vi "Servo.vi"() -> ()   [LabVIEW 2020]
uses:
  <vilib>/MakerHub/LINX/Public/Utilities/Open Serial.vi
  <vilib>/MakerHub/LINX/Public/Sensors/Motion/Servo/Servo Open One Channel.vi
  <vilib>/MakerHub/LINX/Public/Sensors/Motion/Servo/Servo Close One Channel.vi
  <vilib>/MakerHub/LINX/LMH-LINX.lvlib
  <vilib>/MakerHub/LINX/Public/Sensors/Motion/Servo/Servo.lvlib
panel:
  out "Position":dbl
  in  "stop":bool
  in  "Turns":bool
  in  "Servo Channel":u8
  in  "Serial Port":refnum<visa-resource-name>="N/A"
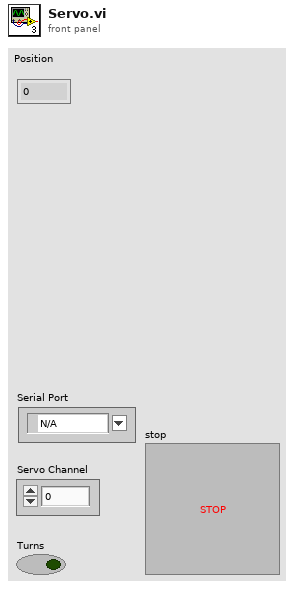
[diagram p1: front panel]
types:
  T1 = typedef "LMH-LINX.lvlib/LINX Ref.ctl" = cluster{"IO":T2, "Interface":T3, "LINX Device Config":T4}
  T2 = typedef "LMH-LINX.lvlib/Platform.ctl" = enum16{"Remote", "Local"}
  T3 = typedef "LMH-LINX.lvlib/Interface.ctl" = enum16{"Serial", "TCP"}
  T4 = typedef "LMH-LINX.lvlib/Device.lvlib/LINX Device Config.ctl" = cluster{"Interface":T3, "COM Port":refnum<visa-resource-name>, "TCP Configuration":T5, "Device Family":u8, "Device ID":u8, "Device Name":string, "TCP Ref":refnum<k5>, "Channels":T6}
  T5 = typedef "LMH-LINX.lvlib/Device.lvlib/TCP Config.ctl" = cluster{"IP Address":string, "Port":u16}
  T6 = typedef "LMH-LINX.lvlib/Channels.ctl" = cluster{"DI":u8[], "DO":u8[], "AI":u8[], "AO":u8[], "PWM":u8[], "QE":u8[], "UART":u8[], "I2C 2":u8[], "SPI":u8[], "CAN":u8[], "Servo":u8[], "AI Ref (V)":dbl, "AI Resolution (Bits)":u8, "AO Ref (V)":dbl, "AO Resolution (Bits)":u8}
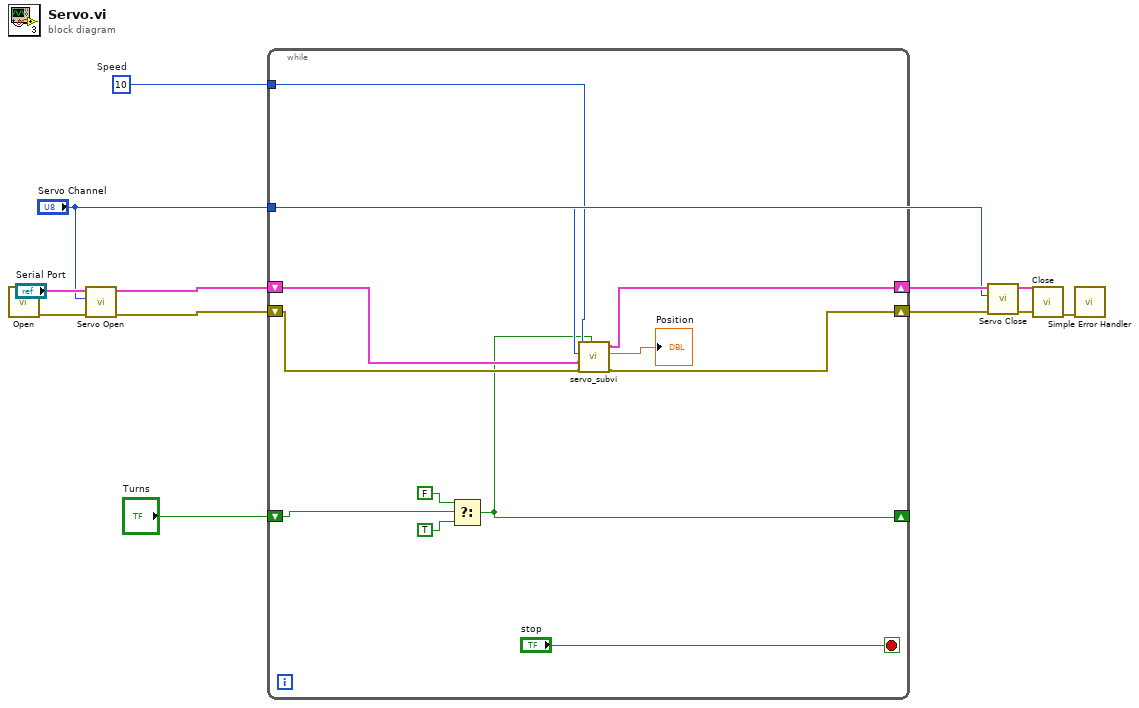
[diagram p0: block diagram]
diagram:
  w1 = u32 10  # Speed
  n1 = call-poly <vilib>:"Open.vi"("Serial Port"="Serial Port") -> ("Error Out"=w11:errorcluster, "LINX Resource"=w12:T1)  [unwired: 8 in, 1 out]
  n2 = call-poly <vilib>:"Servo Open.vi"("Error In"=w11, "Servo Channel"="Servo Channel", "LINX Resource"=w12) -> ("Error Out"=w6:errorcluster, "LINX Resource"=w7:T1)  [unwired: 7 in]
  n3 = while {
    tunnel: "Servo Channel" -> [w21]
    tunnel: w1 -> [w18]
    shift-right: [w22] -> w4
    shift-left: w7 -> [w25]
    shift-right: [w23] -> w5
    shift-left: w6 -> [w24]
    shift-right: [w16] -> _
    shift-left: "Turns" -> [w17]
    stop <- "stop" stop-if-true
    n4 = Select(t=FALSE, s=w17, f=TRUE) -> (s? t:f=w16:bool)
    n5 = call "servo_subvi.vi"("Turns"=w16, "error in (no error)"=w24, "LINX Resource"=w25, "Servo Channel"=w21, "Speed"=w18) -> ("error out"=w23:errorcluster, "Position"=→"Position":dbl, "LINX Resource out"=w22:T1)  [unwired: 3 in]
  }
  n6 = call-poly <vilib>:"Servo Close.vi"("Error In"=w5, "Servo Channel"="Servo Channel", "LINX Resource"=w4) -> ("Error Out"=w9:errorcluster, "LINX Resource"=w10:T1)  [unwired: 7 in]
  n7 = call <vilib>:"Close.vi"("Error In"=w9, "LINX Resource"=w10) -> ("Error Out"=w13:errorcluster)  [unwired: 9 in]
  n8 = call <vilib>:"Simple Error Handler.vi"("error in (no error)"=w13) -> ()  [unwired: 4 in, 5 out]
